vi "Example.vi"() -> ()   [LabVIEW 2022 SP3]
uses:
  <vilib>/MakerHub/LINX/Public/Utilities/Open Serial.vi
  HW-201.lvclass
  <vilib>/MakerHub/LINX/LMH-LINX.lvlib
panel:
  out "Loop Rate (Hz)":u32
  out "Error Out":errorcluster
  out "isOnLine":bool
  in  "Boolean":bool
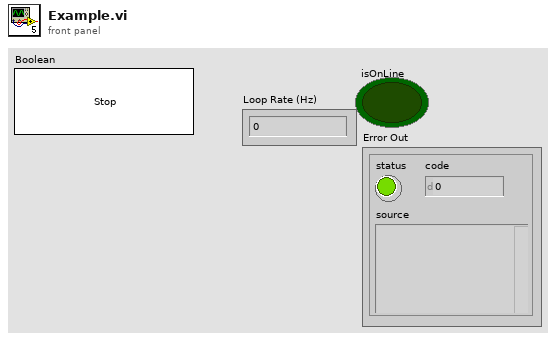
[diagram p1: front panel]
types:
  T1 = typedef "LMH-LINX.lvlib/LINX Ref.ctl" = cluster{"IO":T2, "Interface":T3, "LINX Device Config":T4}
  T2 = typedef "LMH-LINX.lvlib/Platform.ctl" = enum16{"Remote", "Local"}
  T3 = typedef "LMH-LINX.lvlib/Interface.ctl" = enum16{"Serial", "TCP"}
  T4 = typedef "LMH-LINX.lvlib/Device.lvlib/LINX Device Config.ctl" = cluster{"Interface":T3, "COM Port":refnum<visa-resource-name>, "TCP Configuration":T5, "Device Family":u8, "Device ID":u8, "Device Name":string, "TCP Ref":refnum<k5>, "Channels":T6}
  T5 = typedef "LMH-LINX.lvlib/Device.lvlib/TCP Config.ctl" = cluster{"IP Address":string, "Port":u16}
  T6 = typedef "LMH-LINX.lvlib/Channels.ctl" = cluster{"DI":u8[], "DO":u8[], "AI":u8[], "AO":u8[], "PWM":u8[], "QE":u8[], "UART":u8[], "I2C 2":u8[], "SPI":u8[], "CAN":u8[], "Servo":u8[], "AI Ref (V)":dbl, "AI Resolution (Bits)":u8, "AO Ref (V)":dbl, "AO Resolution (Bits)":u8}
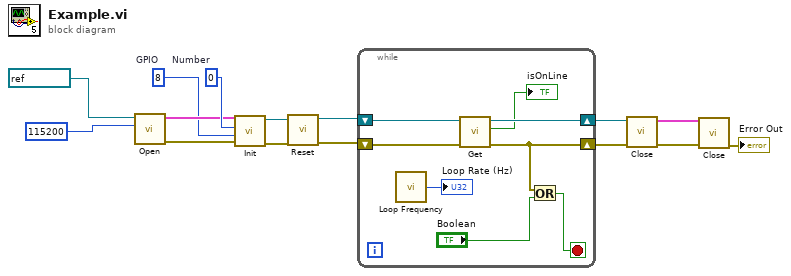
[diagram p0: block diagram]
diagram:
  w13 = u8 0  # Number
  w6 = u8 8  # GPIO
  n1 = call-poly <vilib>:"Open.vi"("Baud Rate Override"=u32 115200, "Serial Port"=refnum<visa-resource-name> "COM5") -> ("Error Out"=w12:errorcluster, "LINX Resource"=w11:T1)  [unwired: 7 in, 1 out]
  n2 = call "Init.vi"("error in (no error)"=w12, "GPIO"=w6, "Number"=w13, "LINX Resource"=w11) -> ("error out"=w4:errorcluster, "HW-201 out"=w3:refnum<class "HW-201.lvclass">)  [unwired: 6 in]
  n3 = call "Reset.vi"("error in (no error)"=w4, "HW-201 in"=w3) -> ("error out"=w1:errorcluster, "HW-201 out"=w2:refnum<class "HW-201.lvclass">)  [unwired: 8 in]
  n4 = while {
    shift-right: [w21] -> w15
    shift-left: w2 -> [w23]
    shift-right: [w18] -> w14
    shift-left: w1 -> [w22]
    stop <- w17 stop-if-true
    n5 = call <vilib>:"Loop Frequency.vi"() -> ("Loop Rate (Hz)"=→"Loop Rate (Hz)":u32)
    n6 = call "Get.vi"("error in (no error)"=w22, "HW-201 in"=w23) -> ("error out"=w18:errorcluster, "isOnLine"=→"isOnLine":bool, "HW-201 out"=w21:refnum<class "HW-201.lvclass">)  [unwired: 7 in]
    n7 = Or(x=w18, y="Boolean") -> (x .or. y?=w17:bool)
  }
  n8 = call <vilib>:"Close.vi"("error in (no error)"=w14, "HW-201 in"=w15) -> ("error out"=w10:errorcluster, "LINX Resource"=w9:T1)  [unwired: 8 in]
  n9 = call <vilib>:"Close.vi"("Error In"=w10, "LINX Resource"=w9) -> ("Error Out"=→"Error Out":errorcluster)  [unwired: 9 in]
